vi "3d (SubVI).vi"(6 "Translation":cluster{"X":sgl, "Y":sgl, "Z":sgl}, 7 "stop":bool, 9 "Axis":cluster{"X":sgl, "Y":sgl, "Z":sgl}, 10 "Angle":sgl(knob) scale=0.0..360.0, 11 "STL File Path":path) -> (0 "error out":errorcluster, 3 "SceneNode out":refnum<vi>(3d-picture))   [LabVIEW 2011]
uses:
  <vilib>/picture/3D Picture Control/NI_3D Picture Control.lvlib
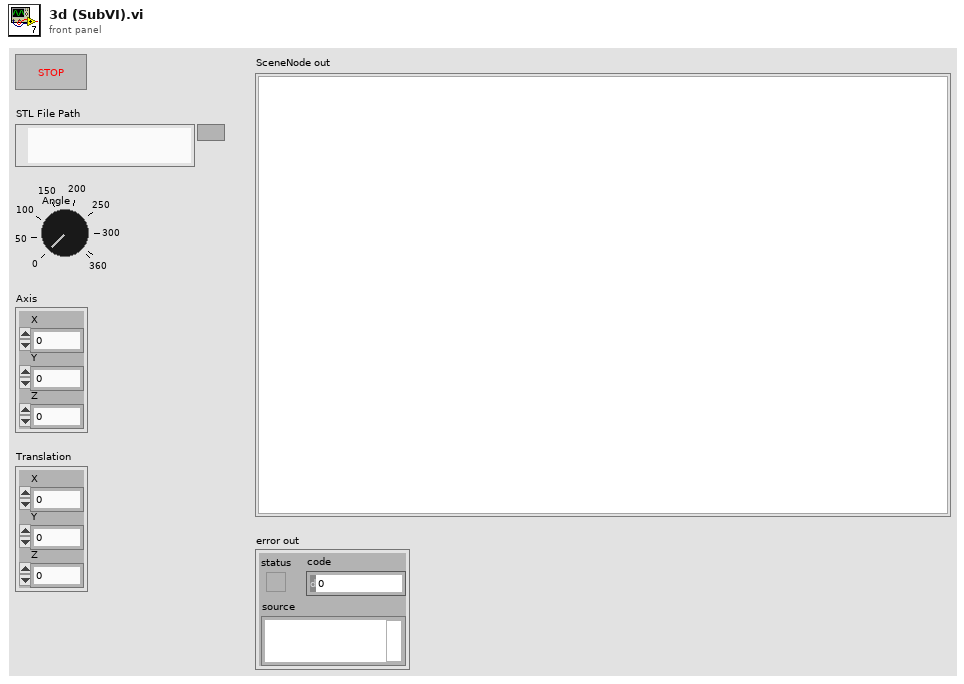
[diagram p1: front panel]
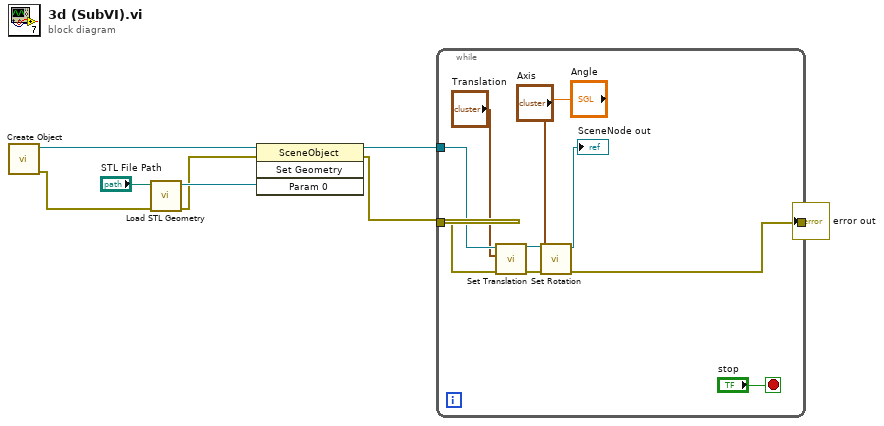
[diagram p0: block diagram]
diagram:
  n1 = call <vilib>:"Create Object.vi"() -> ("error out"=w2:errorcluster, "Scene:New Object"=w3:refnum<vi>)  [unwired: 2 in, 8 out]
  n2 = call <vilib>:"Load STL Geometry.vi"("error in (no error)"=w2, "Model File"="STL File Path") -> ("error out"=w4:errorcluster, "New Mesh Refnum"=w8:refnum<vi>)  [unwired: 8 out]
  n3 = invoke class="SceneObject" method="Set Geometry"(reference=w3, error in=w4, "Param 0"=w8) -> (reference out=w7:refnum<vi>, error out=w5:errorcluster)  [unwired: 1 in, 2 out]
  n4 = while {
    tunnel: w7 -> [w17]
    tunnel: w5 -> [w16]
    tunnel: [w11] -> w6
    stop <- "stop" stop-if-true
    n5 = call <vilib>:"Set Translation.vi"("error in (no error)"=w16, "Translation"="Translation", "Scene Object"=w17) -> ("error out"=w14:errorcluster, "Translated Object"=w13:refnum<vi>)  [unwired: 7 in]
    n6 = call <vilib>:"Set Rotation.vi"("error in (no error)"=w14, "Angle"="Angle", "Axis"="Axis", "Scene Object"=w13) -> ("error out"=w11:errorcluster, "Rotated Scene Object"=→"SceneNode out":refnum<vi>)  [unwired: 6 in]
  }
  "error out" <- w6
